vi "list_folder-advanced.vi"(6 "include_deleted":bool, 8 "error in (no error)":errorcluster, 9 "include_media_info":bool, 10 "recursive":bool, 11 "path":string) -> (0 "error out":errorcluster, 1 "cursor":string, 2 "has_more":bool, 3 "path []":string[](array[string]))   [LabVIEW 2015, in "lv-dropbox.lvlib" / "v2.lvlib"]
uses:
  v2.lvlib
  <vilib>/httpClient/POSTBuffer.vi
  <vilib>/httpClient/LabVIEWHTTPClient.lvlib
  lv-dropbox.lvlib
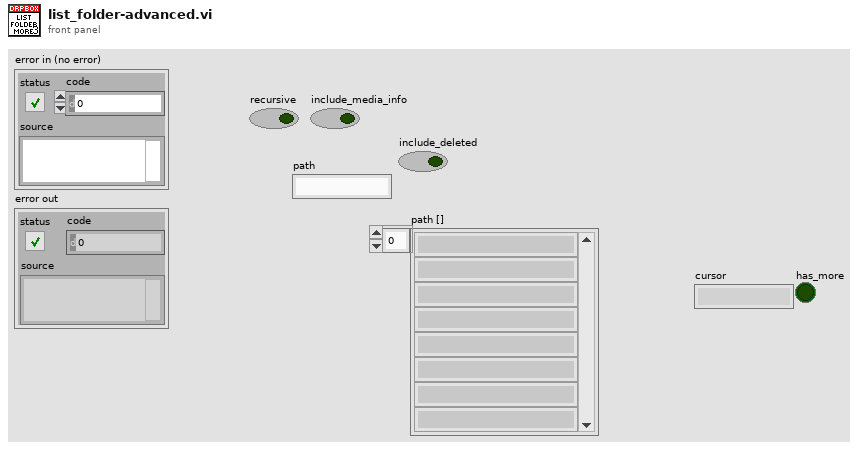
[diagram p1: front panel]
types:
  T1 = cluster{"entries":cluster{".tag":string, "name":string, "path_lower":string, "path_display":string, "id":string}[], "cursor":string, "has_more":bool}
  T2 = cluster{"path":string, "recursive":bool, "include_media_info":bool, "include_deleted":bool}
  T3 = typedef "LabVIEWHTTPClient.lvlib/ClientHandle.ctl" = refnum<k1>
  T4 = cluster{".tag":string, "name":string, "path_lower":string, "path_display":string, "id":string}[]
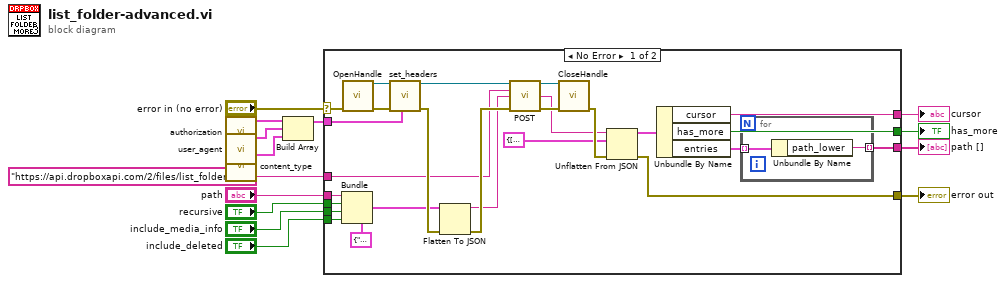
[diagram p0: block diagram]
diagram:
  n1 = call "authorization.vi"() -> ("header"=w5:cluster{"header":string, "value":string})  [unwired: 11 in]
  n2 = call "user_agent.vi"() -> ("header"=w8:cluster{"header":string, "value":string})  [unwired: 11 in]
  n3 = call "content_type.vi"() -> ("header"=w9:cluster{"header":string, "value":string})  [unwired: 11 in]
  n4 = Build Array(w5, w8, w9) -> (w6:cluster{"header":string, "value":string}[])
  n5 = case shown="No Error" "error in (no error)" {
    selector: "error in (no error)" -> [w19 w43]
    tunnel: [w38 w43] -> w14
    tunnel: "include_deleted" -> [w37 _]
    tunnel: "include_media_info" -> [w36 _]
    tunnel: "recursive" -> [w35 _]
    tunnel: "path" -> [w34 _]
    tunnel: "https://api.dropboxapi.com/2/files/list_folder" ("url") -> [w24 _]
    tunnel: w6 -> [w20 _]
    tunnel: [w18 _] -> w3
    tunnel: [w17 _] -> w2
    tunnel: [w16 _] -> w1
    frame No Error {
      n6 = Bundle(cluster=T2 {"path"="", "recursive"=FALSE, "include_media_info"=FALSE, "include_deleted"=FALSE}, "path"=w34, "recursive"=w35, "include_media_info"=w36, "include_deleted"=w37) -> (w31:T2)
      n7 = call <vilib>:"OpenHandle.vi"("error in (no error)"=w19) -> ("client handle out"=w23:T3, "error out"=w21:errorcluster)  [unwired: 13 in]
      n8 = call "set_headers.vi"("header_value []"=w20, "error in (no error)"=w21, "client_handle in"=w23) -> ("error out"=w40:errorcluster, "client_handle out"=w22:T3)  [unwired: 7 in]
      n9 = Flatten To JSON(anything=w31, error in (no error)=w40) -> (JSON string=w30:string, 11:w39:errorcluster)  [unwired: 1 in]
      n10 = call-poly <vilib>:"POST.vi"("client handle"=w22, "url"=w24, "buffer"=w30, "error in (no error)"=w39) -> ("client handle out"=w32:T3, "body"=w28:string, "error out"=w33:errorcluster)  [unwired: 8 in, 1 out]
      n11 = call <vilib>:"CloseHandle.vi"("client handle"=w32, "error in (no error)"=w33) -> ("error out"=w29:errorcluster)  [unwired: 13 in]
      n12 = Unflatten From JSON(JSON string=w28, type and defaults=T1 {"entries"=[], "cursor"="", "has_more"=FALSE}, error in (no error)=w29) -> (value=w27:T1, error out=w38:errorcluster)  [unwired: 4 in]
      n13 = Unbundle By Name(w27) -> ("cursor"=w17:string, "has_more"=w16:bool, "entries"=w26:T4)
      n14 = for {
        tunnel: w26 -> [w42] mode=indexing
        tunnel: [w41] -> w18 mode=indexing
        n15 = Unbundle By Name(w42) -> ("path_lower"=w41:string)
      }
    }
    frame Error {
    }
  }
  "error out" <- w14
  "path []" <- w3
  "cursor" <- w2
  "has_more" <- w1
